vi "_시리얼_Mark10-셋업.vi"(5 "시리얼 포트":refnum<visa-resource-name>="COM5") -> (2 "VISA 리소스 이름 출력":refnum<visa-resource-name>)   [LabVIEW 2015]
panel:
  # "MARK10 게이지 셋업"
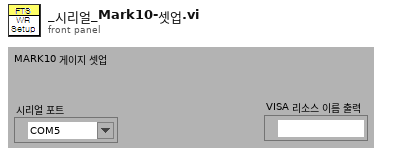
[diagram p1: front panel]
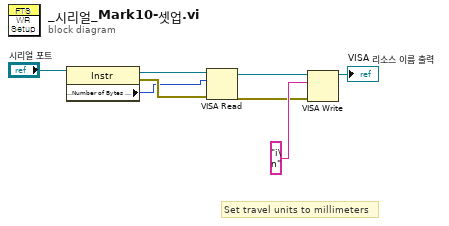
[diagram p0: block diagram]
diagram:
  # "Set travel units to millimeters"
  n1 = property class="Instr"(reference="시리얼 포트") -> (reference out=w7:refnum<visa-resource-name>, error out=w5:errorcluster, "Serial Settings:Number of Bytes at Serial Port"=w2:u32)  [unwired: 1 in]
  n2 = VISA Read(VISA resource name=w7, byte count=w2, error in (no error)=w5) -> (VISA resource name out=w4:refnum<visa-resource-name>, error out=w3:errorcluster)  [unwired: 2 out]
  n3 = VISA Write(VISA resource name=w4, write buffer="i\n", error in (no error)=w3) -> (VISA resource name out=→"VISA 리소스 이름 출력":refnum<visa-resource-name>)  [unwired: 2 out]
